vi "deinitialize.vi"(8 "error in (no error)":errorcluster, 11 "channel (0:all)":u16 format="%x") -> (0 "error out":errorcluster)   [LabVIEW 2024, in "atsj peakcan basic.lvlib"]
doc: "Deinitializes a PeakCAN <b>channel</b>."
uses:
  atsj peakcan basic.lvlib
  support/x64/PCANBasic.dll
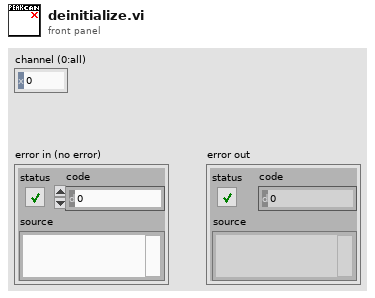
[diagram p1: front panel]
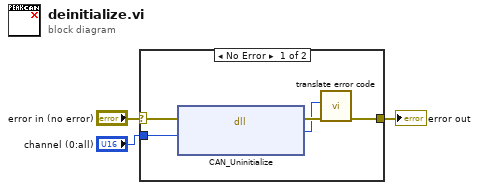
[diagram p0: block diagram]
diagram:
  n1 = case shown="No Error" "error in (no error)" {
    selector: "error in (no error)" -> [w7 w9]
    tunnel: [w5 w9] -> w2
    tunnel: "channel (0:all)" -> [w8 _]
    frame No Error {
      n2 = dll-call lib="C:/atsj/plateau/atsj-peakcan-basic-for-labview/src/support/x64/PCANBasic.dll" fn="CAN_Uninitialize" ("deinitialize")(error in=w7, "Channel"=w8) -> (error out=w6:errorcluster, "Status"=w4:u32)  [unwired: 3 in, 1 out]
      n3 = call "translate error code.vi"("error in (no error)"=w6, "error code"=w4) -> ("error out"=w5:errorcluster)  [unwired: 9 in]
    }
    frame Error {
    }
  }
  "error out" <- w2
